vi "Write FPGA VI Reference.vi"(8 "error in (no error)":errorcluster, 10 "AOD FPGA":T1, 11 "AODAcq in":refnum<class "AODAcq.lvclass">) -> (0 "error out":errorcluster, 3 "AODAcq out":refnum<class "AODAcq.lvclass">)   [LabVIEW 2012, in "AODAcq.lvclass"]
uses:
  AODAcq.lvclass
  FPGA_Control/AODRef.ctl
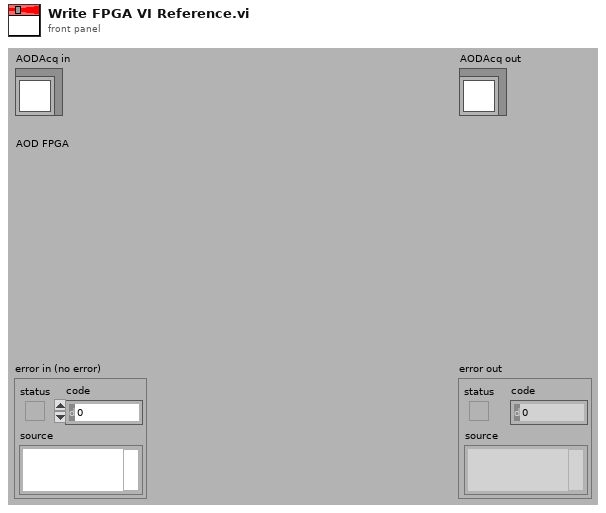
[diagram p1: front panel]
types:
  T1 = typedef "AODRef.ctl" = refnum<k20>
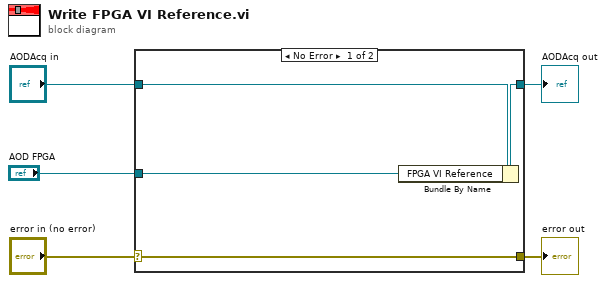
[diagram p0: block diagram]
diagram:
  n1 = case shown="No Error" "error in (no error)" {
    selector: "error in (no error)" -> [w9 w10]
    tunnel: [w9 w10] -> w4
    tunnel: [w7 w11] -> w2
    tunnel: "AODAcq in" -> [w8 w11]
    tunnel: "AOD FPGA" -> [w6 _]
    frame No Error {
      n2 = Bundle By Name(cluster=w8, "FPGA VI Reference"=w6) -> (w7:refnum<class "AODAcq.lvclass">)
    }
    frame Error {
    }
  }
  "error out" <- w4
  "AODAcq out" <- w2
